vi "Page_Source_Get_Inclusion_Types.vi"(8 "error in (no error)":errorcluster, 11 "AB_EXE in":refnum<class "AB_EXE.lvclass">) -> (0 "error out":errorcluster, 2 "supportedFunctions":T1, 3 "AB_EXE out":refnum<class "AB_EXE.lvclass">)   [LabVIEW 2020, in "AB_EXE.lvclass"]
uses:
  <vilib>/AppBuilder/AB_Classes/EXE/AB_EXE.lvclass
  <resource>/Framework/Providers/Builds/AppBuilder/AB_UI_Page_Source_Files_supportedFunctions.ctl
  <vilib>/AppBuilder/AB_Source_Inclusion.ctl
  <vilib>/AppBuilder/AB_Classes/EXE/common/AB_EXE.lvlib
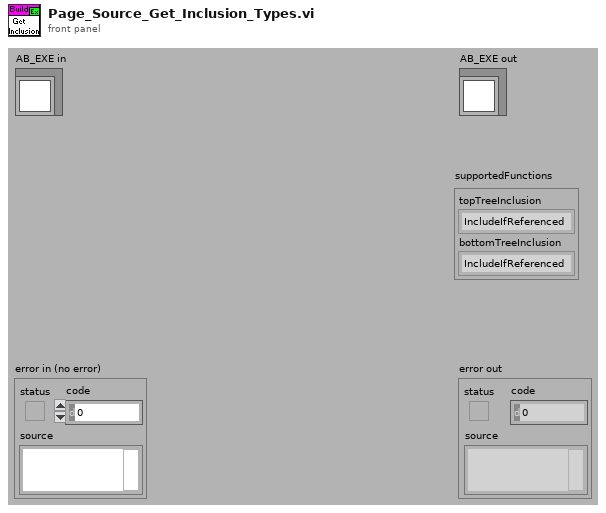
[diagram p1: front panel]
types:
  T1 = typedef "AB_UI_Page_Source_Files_supportedFunctions.ctl" = cluster{"topTreeInclusion":T2, "bottomTreeInclusion":T2}
  T2 = typedef "AB_Source_Inclusion.ctl" = enum16{"IncludeIfReferenced", "Include", "Exclude", "TopLevel"}
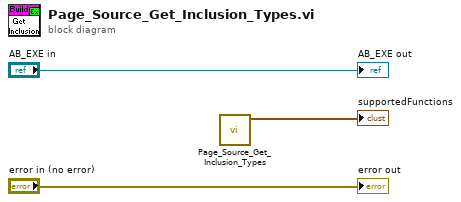
[diagram p0: block diagram]
diagram:
  n1 = call <vilib>:"Page_Source_Get_Inclusion_Types.vi"() -> ("supportedFunctions"=→"supportedFunctions":T1)  [unwired: 11 in]
  "error out" <- "error in (no error)"
  "AB_EXE out" <- "AB_EXE in"
